vi "StimFile-Compute Max Level.vi"(0 "File":T5, 5 "Filter":T3 {"Stages"."IIR Filter"."Forward Coefficients" format="%.4f"; "Stages"."IIR Filter"."Reverse Coefficients" format="%.4f"}, 9 "Level":T1, 11 "error in (no error)":errorcluster, 12 "Sampling Rate (Hz)":dbl, 13 "Npts":i32) -> (6 "Max Level":dbl, 10 "Level out":T1, 15 "error out":errorcluster)   [LabVIEW 2020]
uses:
  StimFile-Params.ctl
  Controls/Advanced Filter XCtl/Filter Data.ctl
  Filter VIs/Filter-Bandwidth Units.ctl
  Controls/Level XCtl/Level Data.ctl
  Controls/Level XCtl/Level Units.ctl
  <vilib>/Analysis/5stat.llb/RMS (DBL).vi
  PXI DAQ VIs/DAQ Engine VIs/PXI Globals.vi
  Utility VIs/Math VIs/Linear to dB (scalar).vi
  <vilib>/Analysis/NI_AALPro.lvlib
  <vilib>/Analysis/2dsp.llb/Inverse Complex FFT.vi
  Controls/Level XCtl/Level XCtl.xctl
  Controls/Advanced Filter XCtl/Advanced Filter XCtl.xctl
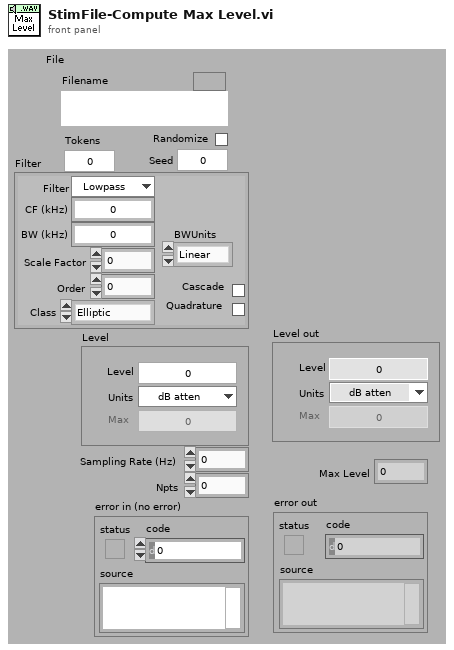
[diagram p1: front panel]
types:
  T1 = typedef "Level XCtl.xctl/Level Data.ctl" = cluster{"Level":dbl, "Units":T2, "Max":dbl, "Multiplier":dbl, "Cal File":path, "Cal":cluster{"Freq (Hz)":dbl[], "Mag (dB SPL)":dbl[], "Phase (deg)":dbl[]}}
  T2 = typedef "Level Units.ctl" = enum16{"dB atten", "dB SPL", "dB re 1 Vrms", "dB V/Hz½", "mW", "dB HL", "Volts", "dB mW"}
  T3 = typedef "Advanced Filter XCtl.xctl/Filter Data.ctl" = cluster{"Type":enum16{"Lowpass", "Highpass", "Bandpass", "Bandstop", "OFF"}, "CF (kHz)":dbl, "BW (kHz)":dbl, "Cascade":bool, "Quadrature":bool, "Scale Factor":dbl, "Stages":cluster{"IIR Filter":cluster{"filter structure":enum32{"IIR 2nd Order", "IIR 4th Order"}, "Reverse Coefficients":dbl[], "Forward Coefficients":dbl[]}, "State":dbl[]}[], "Class":enum16{"Elliptic", "Butterworth"}, "Order":i32, "BWUnits":T4}
  T4 = typedef "Filter-Bandwidth Units.ctl" = enum16{"Linear", "Octaves", "Min-Max"}
  T5 = typedef "StimFile-Params.ctl" = cluster{"Filename":path, "Signal":dbl[], "Channel":i32, "stream":bool, "offset":i32, "nreps":i32, "loops":i32, "Randomize":bool, "order":i32[], "Seed":i32, "Tokens":i32}
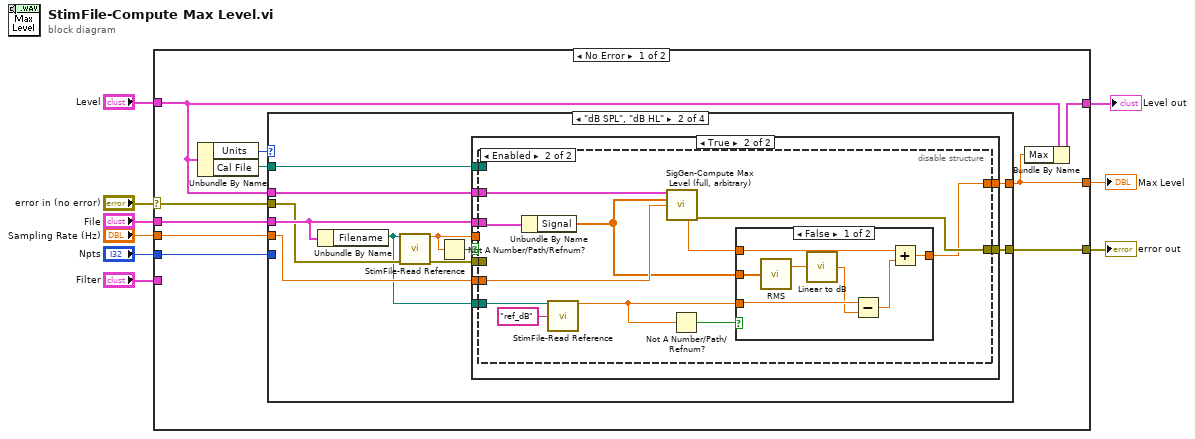
[diagram p0: block diagram]
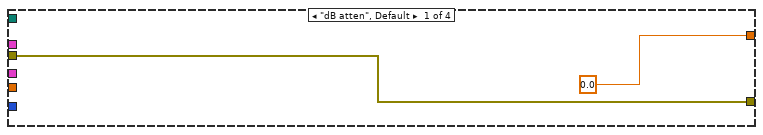
[diagram p2: hidden frame]
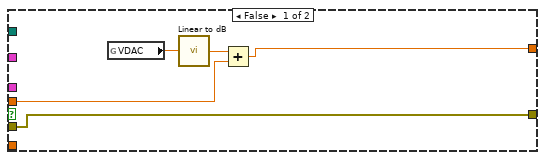
[diagram p3: hidden frame]
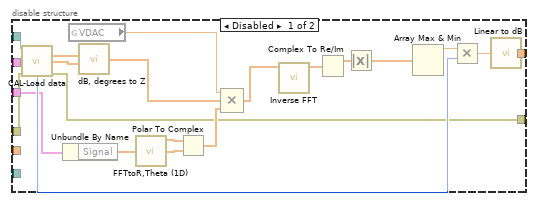
[diagram p4: hidden frame]
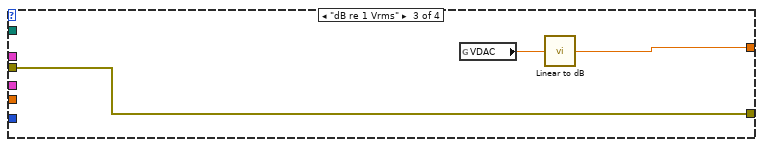
[diagram p6: hidden frame]
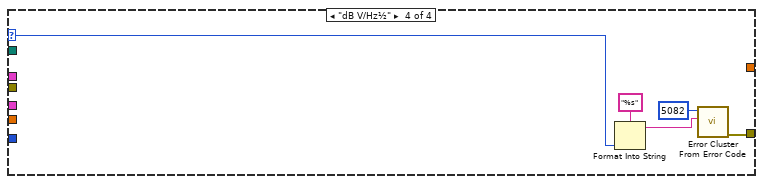
[diagram p7: hidden frame]
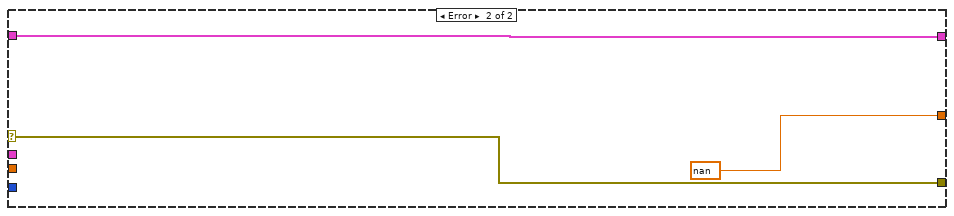
[diagram p8: hidden frame]
diagram:
  n1 = case shown="No Error" "error in (no error)" {
    selector: "error in (no error)" -> [w19 w95]
    tunnel: "Level" -> [w10 w93]
    tunnel: "File" -> [w11 _]
    tunnel: "Filter" -> [_ _]
    tunnel: [w16 w95] -> w8
    tunnel: "Npts" -> [w18 _]
    tunnel: [w15 nan ("Reference Level")] -> w3
    tunnel: "Sampling Rate (Hz)" -> [w17 _]
    tunnel: [w14 w93] -> w1
    frame No Error {
      n2 = Unbundle By Name(w10) -> ("Units"=w13:T2, "Cal File"=w12:path)
      n3 = case shown="\"dB SPL\", \"dB HL\"" w13 {
        selector: w13 -> [_ _ _ w88]
        tunnel: w19 -> [w20 w28 w85 _]
        tunnel: w18 -> [_ _ _ _]
        tunnel: [0.0 ("Reference Level") w31 w86 _] -> w15
        tunnel: w17 -> [_ w24 _ _]
        tunnel: [w20 w30 w85 w89] -> w16
        tunnel: w12 -> [_ w32 _ _]
        tunnel: w11 -> [_ w29 _ _]
        tunnel: w10 -> [_ w23 _ _]
        frame "dB atten", Default {
        }
        frame "dB SPL", "dB HL" {
          n4 = Unbundle By Name(w29) -> ("Filename"=w22:path)
          n5 = call "StimFile-Read Reference.vi"("Wave File"=w22, "error in (no error)"=w28) -> ("Reference (dB)"=w25:dbl, "error out"=w27:errorcluster)  [unwired: 11 in, 1 out]
          n6 = Not A Number/Path/Refnum?(number/path/refnum=w25) -> (NaN/Path/Refnum?=w26:bool)
          n7 = case shown="True" w26 {
            tunnel: w27 -> [w37 w45]
            tunnel: w32 -> [_ w44]
            tunnel: [w33 w43] -> w31
            tunnel: [w37 w39] -> w30
            tunnel: w29 -> [_ w42]
            tunnel: w25 -> [w34 _]
            tunnel: w24 -> [_ w41]
            tunnel: w23 -> [_ w40]
            tunnel: w22 -> [_ w38]
            frame False {
              n8 = global read "PXI Globals.vi" "VDAC"() -> (w36:dbl)
              n9 = call-poly "Linear to dB.vi"("Linear"=w36) -> ("dB"=w35:dbl)
              n10 = Add(x=w35, y=w34) -> (x+y=w33:dbl)
            }
            frame True {
              n11 = disable-structure shown="Enabled" {
                disable-tunnel: w45 -> [w65 _]
                disable-tunnel: w44 -> [w64 _]
                disable-tunnel: [w49 w69] -> w43
                disable-tunnel: w42 -> [w47 w76]
                disable-tunnel: w41 -> [_ w75]
                disable-tunnel: w40 -> [_ w74]
                disable-tunnel: [w48 w73] -> w39
                disable-tunnel: w38 -> [_ w72]
                frame Disabled {
                  n12 = call "CAL-Load data.vi"("user path"=w64, "error in (no error)"=w65) -> ("Mag"=w63:dbl[], "Phase"=w62:dbl[], "npts"=w51:i32, "error out"=w48:errorcluster)  [unwired: 6 in, 4 out]
                  n13 = Unbundle By Name(w47) -> ("Signal"=w46:dbl[])
                  n14 = global read "PXI Globals.vi" "VDAC"() -> (w60:dbl)
                  n15 = call "dB, degrees to Z.vi"("Magnitude (dB)"=w63, "Phase (degrees)"=w62) -> ("Z"=w61:cdb[])  [unwired: 5 in]
                  n16 = call "FFTtoR,Theta (1D).VI"("X"=w46) -> ("+Freq. Mag of FFT"=w58:dbl[], "+Freq Theta of FFT"=w59:dbl[])  [unwired: 1 in]
                  n17 = Polar To Complex(1:w59, 2:w58) -> (0:w57:cdb[])
                  n18 = Compound Arithmetic op=MULTIPLY(w60, w61, w57) -> (w56:cdb[])
                  n19 = call-poly <vilib>:"Inverse FFT.vi"("FFT {X}"=w56) -> ("X"=w55:cdb[])  [unwired: 9 in, 1 out]
                  n20 = Complex To Re/Im(x + iy=w55) -> (x=w54:dbl[])  [unwired: 1 out]
                  n21 = Absolute Value(x=w54) -> (abs(x)=w52:dbl[])
                  n22 = Array Max & Min(array=w52) -> (max value=w53:dbl)  [unwired: 3 out]
                  n23 = Multiply(x=w53, y=w51) -> (x*y=w50:dbl)
                  n24 = call-poly "Linear to dB.vi"("Linear"=w50) -> ("dB"=w49:dbl)
                }
                frame Enabled {
                  n25 = Unbundle By Name(w76) -> ("Signal"=w66:dbl[])
                  n26 = call "StimFile-Read Reference.vi"("Wave File"=w72, "refUnits"="ref_dB") -> ("Reference (dB)"=w67:dbl)  [unwired: 11 in, 2 out]
                  n27 = call "SigGen-Compute Max Level (full, arbitrary).vi"("Level"=w74, "Y"=w66, "Sampling Rate (Hz)"=w75) -> ("Max Level"=w68:dbl, "error out"=w73:errorcluster)  [unwired: 10 in, 1 out]
                  n28 = Not A Number/Path/Refnum?(number/path/refnum=w67) -> (NaN/Path/Refnum?=w70:bool)
                  n29 = case shown="False" w70 {
                    tunnel: [w79 w84] -> w69
                    tunnel: w68 -> [w78 w84]
                    tunnel: w67 -> [w81 _]
                    tunnel: w66 -> [w83 _]
                    frame False {
                      n30 = call-poly <vilib>:"RMS.vi"("X"=w83) -> ("rms value"=w82:dbl)  [unwired: 1 out]
                      n31 = call-poly "Linear to dB.vi"("Linear"=w82) -> ("dB"=w80:dbl)
                      n32 = Subtract(x=w81, y=w80) -> (x-y=w77:dbl)
                      n33 = Add(x=w78, y=w77) -> (x+y=w79:dbl)
                    }
                    frame True {
                    }
                  }
                }
              }
            }
          }
        }
        frame "dB re 1 Vrms" {
          n34 = global read "PXI Globals.vi" "VDAC"() -> (w87:dbl)
          n35 = call-poly "Linear to dB.vi"("Linear"=w87) -> ("dB"=w86:dbl)
        }
        frame "dB V/Hz½" {
          n36 = Format Into String(format string="%s", w88) -> (resulting string=w91:string)  [unwired: 2 in, 1 out]
          n37 = call <vilib>:"Error Cluster From Error Code.vi"("error message (\"\")"=w91, "error code (0)"=5082) -> ("error out"=w89:errorcluster)  [unwired: 7 in]
        }
      }
      n38 = Bundle By Name(cluster=w10, "Max"=w15) -> (w14:T1)
    }
    frame Error {
    }
  }
  "error out" <- w8
  "Max Level" <- w3
  "Level out" <- w1
